vi "Set Theme Font.vi"(8 "error in (no error)":errorcluster, 10 "Properties:Font":T1, 11 "Filled Text Fields in":refnum<class "Filled Text Fields.lvclass">) -> (0 "error out":errorcluster, 3 "Filled Text Fields out":refnum<class "Filled Text Fields.lvclass">)   [LabVIEW 2017, in "Filled Text Fields Actor.lvlib" / "Filled Text Fields.lvclass"]
uses:
  Filled Text Fields.lvclass
  Theme/Theme.Font/Font.ctl
  Filled Text Fields.lvclass/Filled Text Fields.ctl
  Theme/Theme/setFont.vi
  Theme/Theme/Theme.lvclass
  Filled Text Fields Actor Messages/onDisplayStateChange Msg/onDisplayStateChange Msg.lvclass
  Theme/Theme.Font/Theme.Font.lvclass
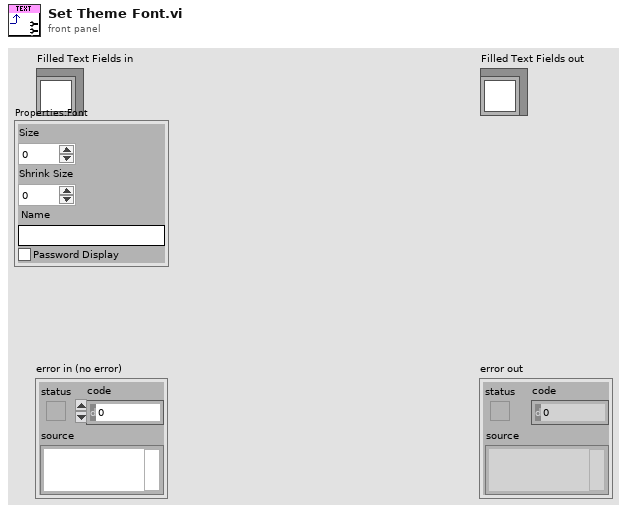
[diagram p1: front panel]
types:
  T1 = typedef "Theme.lvlib/Theme.Font.lvclass/Font.ctl" = cluster{"Size":u32, "Shrink Size":u32, "Name":string, "Password Display":bool}
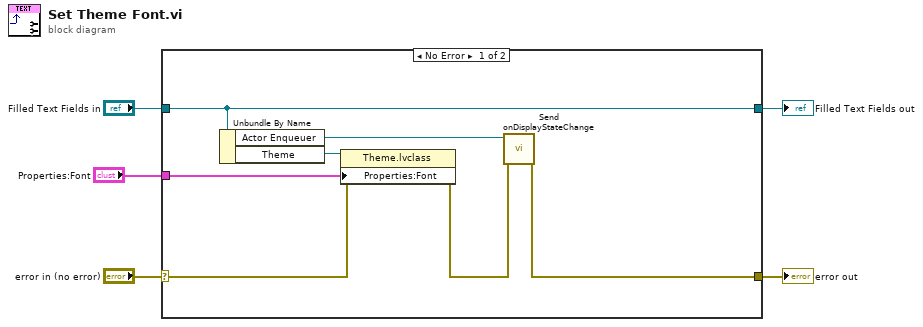
[diagram p0: block diagram]
diagram:
  n1 = case shown="No Error" "error in (no error)" {
    selector: "error in (no error)" -> [w10 w14]
    tunnel: [w6 w14] -> w4
    tunnel: [w12 w13] -> w2
    tunnel: "Filled Text Fields in" -> [w12 w13]
    tunnel: "Properties:Font" -> [w9 _]
    frame No Error {
      n2 = Unbundle By Name(w12) -> ("Actor Enqueuer"=w8:refnum<class "Message Enqueuer.lvclass">, "Theme"=w11:refnum<class "Theme.lvclass">)
      n3 = property class="Theme.lvclass"(reference=w11, error in=w10, "Properties:Font"=w9) -> (error out=w7:errorcluster)  [unwired: 1 out]
      n4 = call "Send onDisplayStateChange.vi"("error in (no error)"=w7, "Message Enqueuer in"=w8) -> ("error out"=w6:errorcluster)  [unwired: 8 in, 1 out]
    }
    frame Error {
    }
  }
  "error out" <- w4
  "Filled Text Fields out" <- w2
